vi "Sub Max Bits.vi"(8 "error in (no error)":errorcluster, 10 "Count":i32, 11 "Packet in":refnum<class "Packet.lvclass">) -> (0 "error out":errorcluster, 3 "Packet out":refnum<class "Packet.lvclass">)   [LabVIEW 2020, in "Packet.lvclass"]
uses:
  Packet.lvclass
  Packet.lvclass/Packet.ctl
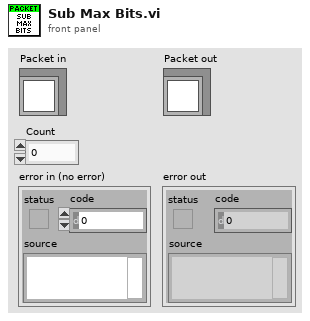
[diagram p1: front panel]
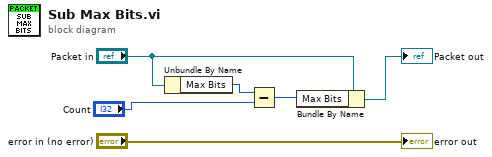
[diagram p0: block diagram]
diagram:
  n1 = Unbundle By Name("Packet in") -> ("Max Bits"=w5:i32)
  n2 = Subtract(x=w5, y="Count") -> (x-y=w3:i32)
  n3 = Bundle By Name(cluster="Packet in", "Max Bits"=w3) -> (→"Packet out":refnum<class "Packet.lvclass">)
  "error out" <- "error in (no error)"
